vi "Get Item Type.vi"(8 "error in (no error)":errorcluster, 9 "Tag":string, 11 "TreeControl in":refnum<vi>) -> (0 "error out":errorcluster, 2 "Item Type":T1=enum."Channel", 3 "TreeControl out":refnum<vi>)   [LabVIEW 2020, in "DSF Core.lvlib"]
uses:
  DSF Core.lvlib
  ID to Tree Items/Tree Item Type.ctl
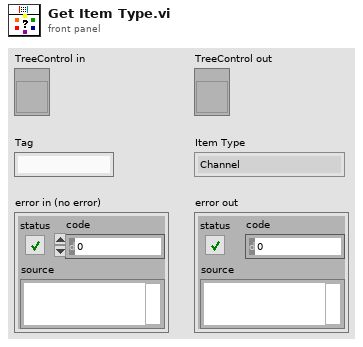
[diagram p1: front panel]
types:
  T1 = typedef "DSF Core.lvlib/Tree Item Type.ctl" = enum16{"Framework", "Plugin Group", "Plugin", "Group", "Transfer", "Buffer", "Channel"}
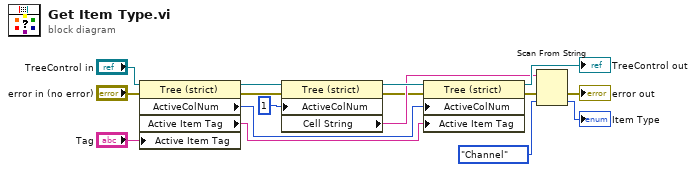
[diagram p0: block diagram]
diagram:
  n1 = property class="Tree (strict)"(reference="TreeControl in", error in="error in (no error)", "Active Item Tag"="Tag") -> (reference out=w10:refnum<vi>, error out=w13:errorcluster, "ActiveColNum"=w12:i32, "Active Item Tag"=w1:string)
  n2 = property class="Tree (strict)"(reference=w10, error in=w13, "ActiveColNum"=1 ("Active Cell:Active Column Number")) -> (reference out=w11:refnum<vi>, error out=w3:errorcluster, "Cell String"=w8:string)
  n3 = property class="Tree (strict)"(reference=w11, error in=w3, "ActiveColNum"=w12, "Active Item Tag"=w1) -> (reference out=→"TreeControl out":refnum<vi>, error out=w5:errorcluster)
  n4 = Scan From String(input string=w8, error in=w5, default 1=Tree_Item_Type."Channel" ("Item Type")) -> (error out=→"error out":errorcluster, output 1=→"Item Type":T1)  [unwired: 2 in, 2 out]
